vi "Read Pressure Transducers.vi"(8 "Error In":errorcluster, 10 "tdms file":refnum<k34>, 11 "task in":refnum<k21>) -> (0 "Error Out":errorcluster, 1 "Tube Pressure":dbl[unit], 2 "Manifold Pressure":dbl[unit], 3 "task out":refnum<k21>, 4 "Readings":T1, 6 "Calibration coefficients":T2)   [LabVIEW 2018]
uses:
  <vilib>/DAQmx/read.llb/DAQmx Read.vi
  <vilib>/DAQmx/read.llb/DAQmx Read (Analog 1D DBL NChan 1Samp).vi
  <vilib>/DAQmx/miscellaneous.llb/DAQmx Fill In Error Info.vi
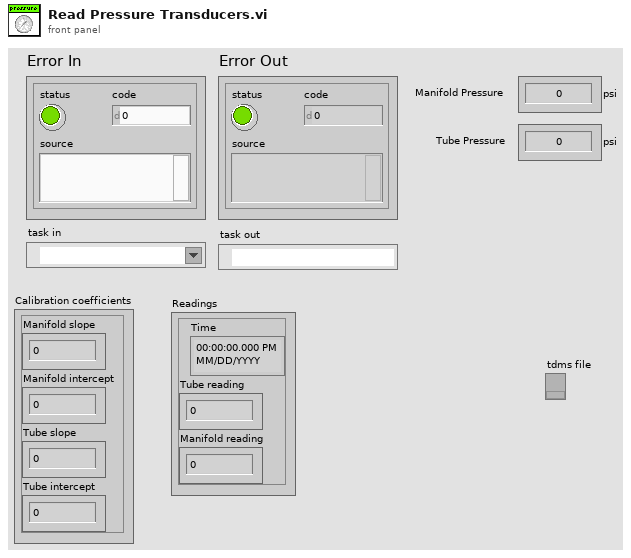
[diagram p1: front panel]
types:
  T1 = cluster{"Time":timestamp, "Tube reading":dbl, "Manifold reading":dbl}
  T2 = cluster{"Manifold slope":dbl, "Manifold intercept":dbl, "Tube slope":dbl, "Tube intercept":dbl}
  T3 = cluster{"Manifold slope":dbl, "Manifold intercept":dbl, "Tube slope":dbl, dbl}
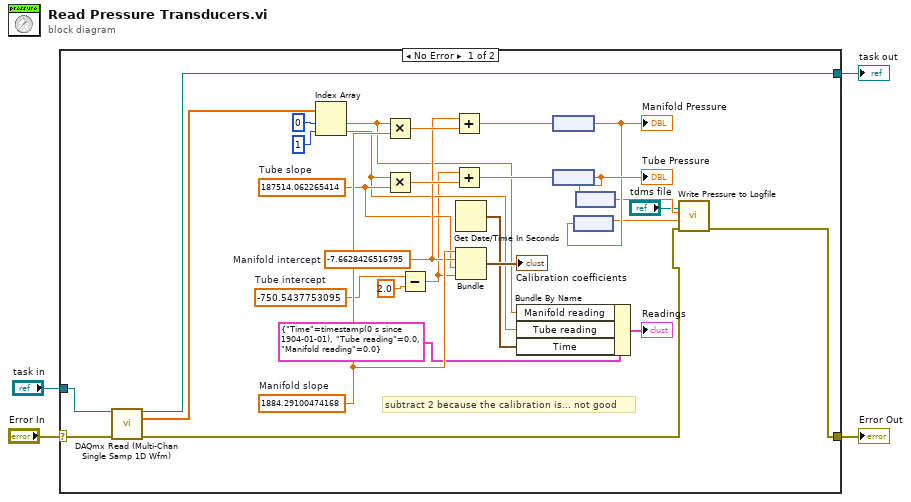
[diagram p0: block diagram]
diagram:
  n1 = case shown="No Error" "Error In" {
    selector: "Error In" -> [w31 w35]
    tunnel: [w6 w35] -> w3
    tunnel: "task in" -> [w32 w34]
    tunnel: [w30 w34] -> w1
    frame No Error {
      w13 = -750.5437753095  # Tube intercept
      w20 = 187514.062265414  # Tube slope
      w21 = -7.6628426516795  # Manifold intercept
      w22 = 1884.29100474168  # Manifold slope
      # "subtract 2 because the calibration is... not good"
      n2 = call-poly "DAQmx Read (Multi-Chan Single Samp 1D Wfm).vi"("task/channels in"=w32, "error in"=w31) -> ("task out"=w30:refnum<k21>, "data"=w33:dbl[], "error out"=w29:errorcluster)  [unwired: 11 in]
      n3 = Index Array(array=w33, index #1=0 ("index"), index #2=1 ("index")) -> (element #1=w18:dbl, element #2=w17:dbl)
      n4 = Multiply(x=w18, y=w22) -> (x*y=w26:dbl)
      n5 = Multiply(x=w17, y=w20) -> (x*y=w24:dbl)
      n6 = Subtract(x=w13, y=2.0) -> (x-y=w11:dbl)
      n7 = Add(x=w21, y=w26) -> (x+y=w25:dbl)
      n8 = Add(x=w11, y=w24) -> (x+y=w23:dbl)
      n9 = Get Date/Time In Seconds() -> (seconds since 1Jan1904=w15:timestamp)
      n10 = Bundle("Manifold slope"=w22, "Manifold intercept"=w21, "Tube slope"=w20, w11) -> (→"Calibration coefficients":T3)  [unwired: 1 in]
      n11 = Bundle By Name(cluster=T1 {"Time"=timestamp(0 s since 1904-01-01), "Tube reading"=0.0, "Manifold reading"=0.0} ("input cluster"), "Manifold reading"=w18, "Tube reading"=w17, "Time"=w15) -> (→"Readings":T1)
      n12 = node(w25) -> (w9:dbl[unit])
      "Manifold Pressure" <- w9
      n13 = node(w23) -> (w10:dbl[unit])
      "Tube Pressure" <- w10
      n14 = node(w9) -> (w7:dbl)
      n15 = node(w10) -> (w8:dbl)
      n16 = call "Write Pressure to Logfile.vi"("error in (no error)"=w29, "Manifold Pressure (Pa)"=w7, "Tube Pressure (Pa)"=w8, "tdms file"="tdms file") -> ("error out"=w6:errorcluster)  [unwired: 6 in, 1 out]
    }
    frame Error {
    }
  }
  "Error Out" <- w3
  "task out" <- w1
